vi "Compute Convolution Rotated Components.vi"(8 "Error In":errorcluster, 9 "Period":dbl, 10 "Step":dbl, 11 "Plot":T1) -> (0 "Error Out":errorcluster, 3 "Convolution Kernels":dbl[][](array[numeric]))   [LabVIEW 2021, in "Fits.lvlib"]
uses:
  Fits.lvlib
  Graphs/XY Graph/XY Plot Data.ctl
  dd787d19-cd8e-4e4e-9265-928e1ec7d284.vi
  3207ea81-9877-4d71-a524-686c1238b2f9.vi
  06af934a-d602-4465-b0be-89c3cfaa1b53.vi
  <vilib>/Utility/error.llb/Error Cluster From Error Code.vi
  Graphs/XY Graph/XY Graph Add-Ons.lvlib
  819f79b2-0da5-4640-b1ec-ec9ad3774aa0.vi
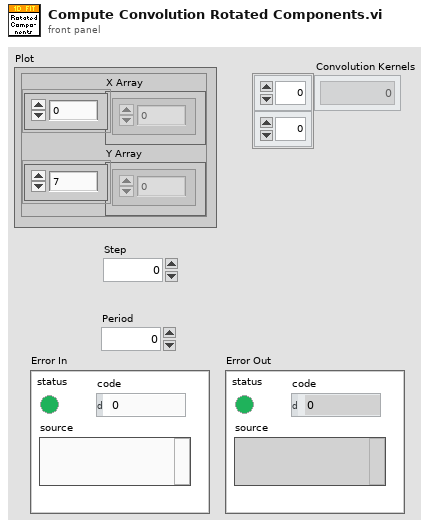
[diagram p1: front panel]
types:
  T1 = typedef "XY Graph Add-Ons.lvlib/XY Plot Data.ctl" = cluster{"X Array":dbl[], "Y Array":dbl[]}
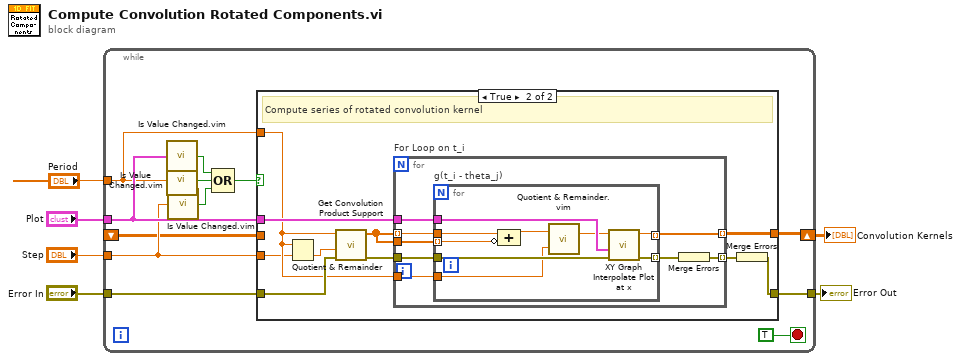
[diagram p0: block diagram]
diagram:
  n1 = while {
    tunnel: "Plot" -> [w16]
    tunnel: "Period" -> [w15]
    tunnel: "Step" -> [w14]
    tunnel: "Error In" -> [w18]
    tunnel: [w17] -> w5
    shift-right: [w8] -> w1
    shift-left: _ -> [w7]
    stop <- TRUE stop-if-true
    n2 = call "Is Value Changed.vim"("value"=w16) -> ("changed or first call?"=w12:bool)
    n3 = call "Is Value Changed.vim"("value"=w15) -> ("changed or first call?"=w13:bool)
    n4 = call "Is Value Changed.vim"("value"=w14) -> ("changed or first call?"=w11:bool)
    n5 = Compound Arithmetic op=OR(w12, w13, w11) -> (w10:bool)
    n6 = case shown="True" w10 {
      tunnel: w18 -> [w20 w29]
      tunnel: [w20 w28] -> w17
      tunnel: w16 -> [_ w24]
      tunnel: w15 -> [_ w23]
      tunnel: w14 -> [_ w22]
      tunnel: [w19 w21] -> w8
      tunnel: w7 -> [w19 _]
      frame False {
      }
      frame True {
        # "Compute series of rotated convolution kernel"
        n7 = Quotient & Remainder(x=w23, y=w22) -> (floor(x/y)=w30:dbl)  [unwired: 1 out]
        n8 = call "Get Convolution Product Support.vi"("Error In"=w29, "# Values"=w30, "IRF Period"=w23) -> ("Error Out"=w25:errorcluster, "Ramp"=w26:dbl[])  [unwired: 6 in, 1 out]
        n9 = for "For Loop on t_i" {
          tunnel: w26 -> [w38] mode=indexing
          tunnel: w26 -> [w34]
          tunnel: [w31] -> w21 mode=indexing
          tunnel: w25 -> [w37]
          tunnel: [w35] -> w27 mode=indexing
          tunnel: w24 -> [w33]
          tunnel: w23 -> [w32]
          n10 = for "g(t_i - theta_j)" {
            tunnel: w38 -> [w47]
            tunnel: [w46] -> w31 mode=indexing
            tunnel: w34 -> [w45] mode=indexing
            tunnel: w37 -> [w44]
            tunnel: [w43] -> w36 mode=indexing
            tunnel: w33 -> [w42]
            tunnel: w32 -> [w40]
            n11 = Compound Arithmetic op=ADD(w47, invert w45) -> (w41:dbl)
            n12 = call "Quotient & Remainder.vim"("y"=w40, "x"=w41) -> ("x - E(x/y)y"=w39:dbl)  [unwired: 1 out]
            n13 = call "XY Graph Interpolate Plot at x.vi"("Error In"=w44, "XY Plot"=w42, "t"=w39) -> ("Error Out"=w43:errorcluster, "XY Plot(t)"=w46:dbl)  [unwired: 7 in]
          }
          n14 = Merge Errors(w36) -> (w35:errorcluster)
        }
        n15 = Merge Errors(w27) -> (w28:errorcluster)
      }
    }
  }
  "Error Out" <- w5
  "Convolution Kernels" <- w1
